vi "Start const speed move.vi"(0 "Zaber":T1={"Serial port handle"="", "Axis"="", "Controller #"=0, "Min position"=0.0, "Max position"=0.0, "Min velocity"=0.0, "Max velocity"=0.0, "Firmware"="", "Device ID"=0, "Variable event"=refnum, "Variable ref"=refnum, "Resolution, usteps/step"=0, "Serial port semaphore"=refnum, "Joystick buttons"={"MinDir"=1, "MaxDir"=2, "MedSpeed"=5, "HighSpeed"=6}} {"Joystick buttons"."HighSpeed" min=1 max=25 step=1; "Joystick buttons"."MedSpeed" min=1 max=25 step=1; "Joystick buttons"."MaxDir" min=1 max=25 step=1; "Joystick buttons"."MinDir" min=1 max=25 step=1}, 2 "Velocity, mm/s":dbl, 5 "error in":errorcluster) -> (14 "Zaber out":T1={"Serial port handle"="", "Axis"="", "Controller #"=0, "Min position"=0.0, "Max position"=0.0, "Min velocity"=0.0, "Max velocity"=0.0, "Firmware"="", "Device ID"=0, "Variable event"=refnum, "Variable ref"=refnum, "Resolution, usteps/step"=0, "Serial port semaphore"=refnum, "Joystick buttons"={"MinDir"=1, "MaxDir"=2, "MedSpeed"=5, "HighSpeed"=6}} {"Joystick buttons"."HighSpeed" min=1 max=25 step=1; "Joystick buttons"."MedSpeed" min=1 max=25 step=1; "Joystick buttons"."MaxDir" min=1 max=25 step=1; "Joystick buttons"."MinDir" min=1 max=25 step=1}, 16 "Velocity, mm/s":dbl, 19 "error out":errorcluster)   [LabVIEW 2017]
uses:
  CommandZaber.ctl
  GenericDataEvent/GenericData.ctl
  GenericDataEvent/GenericEvent.ctl
  Zaber.ctl
  ZaberVariables.ctl
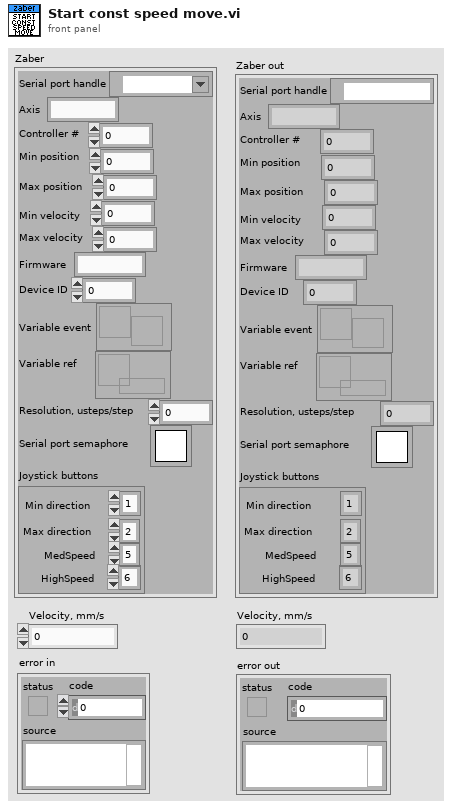
[diagram p1: front panel]
types:
  T1 = typedef "Zaber.ctl" = cluster{"Serial port handle":refnum<visa-resource-name>, "Axis":string, "Controller #":u8, "Min position":dbl, "Max position":dbl, "Min velocity":dbl, "Max velocity":dbl, "Firmware":string, "Device ID":i32, "Variable event":T2, "Variable ref":refnum<data-value>, "Resolution, usteps/step":i32, "Serial port semaphore":T3, "Joystick buttons":cluster{"MinDir":i32, "MaxDir":i32, "MedSpeed":i32, "HighSpeed":i32}}
  T2 = typedef "GenericEvent.ctl" = refnum<user-event>
  T3 = typedef "Semaphore RefNum" = refnum<k1>
  T4 = typedef "CommandZaber.ctl" = cluster{"Command":u8, "Data":i32}
  T5 = typedef "ZaberVariables.ctl" = cluster{"Position":i32, "Speed":i32, "Min soft position":dbl, "Max soft position":dbl, "Accelaration":i32}
  T6 = typedef "GenericData.ctl" = cluster{"Name":string, "Data":variant}
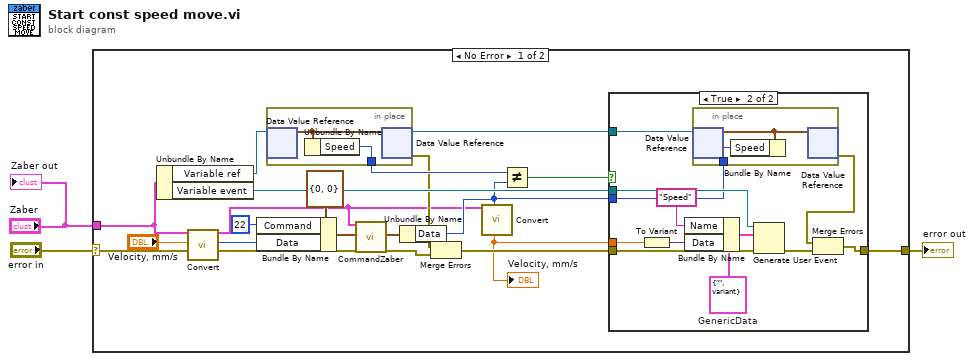
[diagram p0: block diagram]
diagram:
  n1 = case shown="No Error" "error in" {
    selector: "error in" -> [w20 w41]
    tunnel: [w18 w41] -> w2
    tunnel: "Zaber" -> [w5 _]
    frame No Error {
      n2 = Unbundle By Name(w5) -> ("Variable ref"=w16:refnum<data-value>, "Variable event"=w17:T2)
      n3 = call "Convert.vi"("Zaber"=w5, "Velocity, mm/s"="Velocity, mm/s") -> ("Zaber out"=w4:T1, "Velocity, counts"=w7:i32)  [unwired: 9 in, 7 out]
      n4 = Bundle By Name(cluster=T4 {"Command"=0, "Data"=0} ("Command"), "Command"=u8 22, "Data"=w7) -> (w21:T4)
      n5 = in-place {
        in-place-border: [w39] -> w14
        n6 = in-place-dvr #1(w16) -> (w40:T5)  [unwired: 1 out]
        n7 = Unbundle By Name(w40) -> ("Speed"=w39:i32)
        n8 = in-place-dvr #1(w40) -> (w13:refnum<data-value>, w10:errorcluster)
      }
      n9 = call "CommandZaber.vi"("Zaber"=w4, "Command"=w21, "error in"=w20) -> ("Answer"=w19:T4, "error out"=w12:errorcluster)  [unwired: 13 in, 2 out]
      n10 = Unbundle By Name(w19) -> ("Data"=w6:i32)
      n11 = Merge Errors(w10, w12) -> (w11:errorcluster)
      n12 = call "Convert.vi"("Zaber"=w4, "Velocity, counts"=w6) -> ("Velocity, mm/s"=w9:dbl)  [unwired: 9 in, 8 out]
      "Velocity, mm/s" <- w9
      n13 = Not Equal?(x=w14, y=w6) -> (x != y?=w15:bool)
      n14 = case shown="True" w15 {
        tunnel: [w24 w26] -> w18
        tunnel: w9 -> [_ w36]
        tunnel: w11 -> [w24 w35]
        tunnel: w17 -> [_ w31]
        tunnel: w6 -> [_ w28]
        tunnel: w13 -> [_ w29]
        frame False {
        }
        frame True {
          w34 = T6 {"Name"="", "Data"=variant}  # GenericData
          n15 = To Variant(anything=w36) -> (Variant=w30:variant)
          n16 = Bundle By Name(cluster=w34, "Name"="Speed", "Data"=w30) -> (w32:T6)
          n17 = in-place {
            in-place-border: w28 -> [w37]
            n18 = in-place-dvr #2(w29) -> (w38:T5)  [unwired: 1 out]
            n19 = Bundle By Name(cluster=w38, "Speed"=w37) -> ()  [unwired: 1 out]
            n20 = in-place-dvr #2(w38) -> (w25:errorcluster)  [unwired: 1 out]
          }
          n21 = Generate User Event(user event=w31, event data cluster=w32, error in=w35) -> (error out=w27:errorcluster)  [unwired: 1 in, 1 out]
          n22 = Merge Errors(w25, w27) -> (w26:errorcluster)
        }
      }
    }
    frame Error {
    }
  }
  "error out" <- w2
  "Zaber out" <- "Zaber"
